vi "Get Target Virt Instrs.vi"(11 "Measure and Stimulus Subsystems in":refnum<class "Measure and Stimulus Subsystems.lvclass">) -> (2 "Target Virt Instrs":string[](array[string]), 3 "Measure and Stimulus Subsystems out":refnum<class "Measure and Stimulus Subsystems.lvclass">)   [LabVIEW 2023, in "HAL GOOP4.lvlib" / "Measure and Stimulus Subsystems.lvclass"]
uses:
  Measure and Stimulus Subsystems.lvclass
  Measure and Stimulus Subsystems.lvclass/Measure and Stimulus Subsystems.ctl
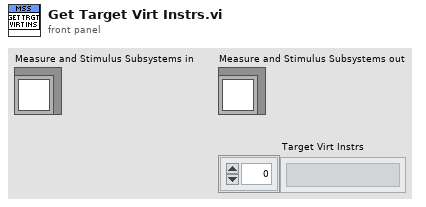
[diagram p1: front panel]
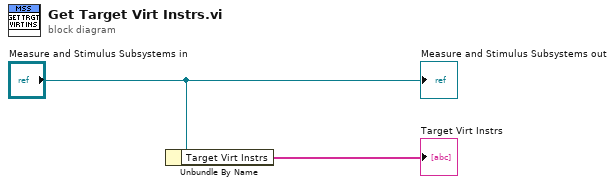
[diagram p0: block diagram]
diagram:
  n1 = Unbundle By Name("Measure and Stimulus Subsystems in") -> ("Target Virt Instrs"=→"Target Virt Instrs":string[])
  "Measure and Stimulus Subsystems out" <- "Measure and Stimulus Subsystems in"
